vi "saveAsDocument.vi"(8 "error in (no error)":errorcluster, 10 "File Path":path, 11 "MS-Word in":refnum<class "MS-Word.lvclass">) -> (0 "error out":errorcluster, 3 "MS-Word out":refnum<class "MS-Word.lvclass">)   [LabVIEW 2017, in "LabVIEW NPOI.lvlib" / "MS-Word.lvclass"]
doc: "Protected dynamic dispatch method to save the <b>Document</b> to the given <b>File Path</b>."
uses:
  MS-Word.lvclass
  MS-Word.lvclass/MS-Word.ctl
  xwpfWriter/xwpfWriter.lvclass
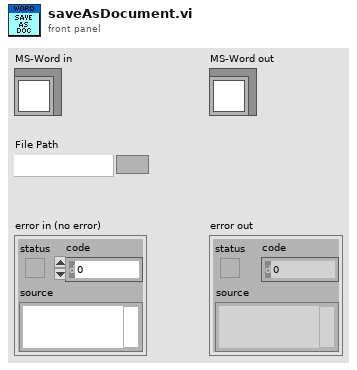
[diagram p1: front panel]
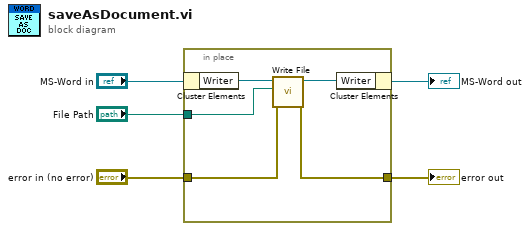
[diagram p0: block diagram]
diagram:
  n1 = in-place {
    in-place-border: "File Path" -> [w8]
    in-place-border: "error in (no error)" -> [w7]
    in-place-border: [w6] -> w1
    n2 = in-place-cluster #1("MS-Word in") -> ("Writer"=w10:refnum<class "xwpfWriter.lvclass">)
    n3 = call "Write File.vi"("error in (no error)"=w7, "path"=w8, "xwpfWriter in"=w10) -> ("error out"=w6:errorcluster, "xwpfWriter out"=w9:refnum<class "xwpfWriter.lvclass">)  [unwired: 7 in]
    n4 = in-place-cluster #1("Writer"=w9) -> (→"MS-Word out":refnum<class "MS-Word.lvclass">)
  }
  "error out" <- w1
